vi "ArmMotorControl.vi"(2 "InputWhenFalse":dbl, 3 "EncoderDistance":dbl) -> ()   [LabVIEW 2018]
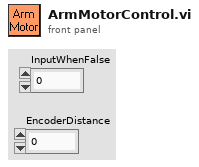
[diagram p1: front panel]
types:
  T1 = typedef "WPI_MotorControlDeviceRef.ctl" = cluster{"DeviceStatus":errorcluster, "Type":T2, "PWM":cluster{"PWM Channel":T3, "DeadBand":T4}, "CAN":cluster{"Device Number":u8, "SetOutput VI Ref":variant, "GetOutput VI Ref":variant, "Enable VI Ref":variant, "Disable VI Ref":variant, "Data":variant}, "Invert":bool, "DIO PWM":cluster{"PWM \"Enable\" Channel":T3, "DIOChannel":T5, "PWM Rate":dbl}}
  T2 = typedef "WPI_MotorControlType.ctl" = enum16{"PWM", "CAN", "DIO PWM"}
  T3 = typedef "FPGA_DIOPWMChannel.ctl" = enum8{"PWM 0", "PWM 1", "PWM 2", "PWM 3", "PWM 4", "PWM 5", "PWM 6", "PWM 7", "PWM 8", "PWM 9", "PWM MXP 0", "PWM MXP 1", "PWM MXP 2", "PWM MXP 3", "PWM MXP 4", "PWM MXP 5", "PWM MXP 6", "PWM MXP 7", "PWM MXP 8", "PWM MXP 9", "Invalid"}
  T4 = typedef "WPI_PWMDeadband.ctl" = cluster{"Name":string, "maxPositivePwm":i32, "minPositivePwm":i32, "centerPwm":i32, "maxNegativePwm":i32, "minNegativePwm":i32, "angularRange":u16}
  T5 = typedef "FPGA_DIOChannel.ctl" = enum8{"DIO 0", "DIO 1", "DIO 2", "DIO 3", "DIO 4", "DIO 5", "DIO 6", "DIO 7", "DIO 8", "DIO 9", "DIO MXP 0", "DIO MXP 1", "DIO MXP 2", "DIO MXP 3", "DIO MXP 4", "DIO MXP 5", "DIO MXP 6", "DIO MXP 7", "DIO MXP 8", "DIO MXP 9", "DIO MXP 10", "DIO MXP 11", "DIO MXP 12", "DIO MXP 13", "DIO MXP 14", "DIO MXP 15", "SPI Port CS1", "SPI Port CS2", "SPI Port CS3", "SPI Port MISO", "SPI Port MOSI", "Invalid"}
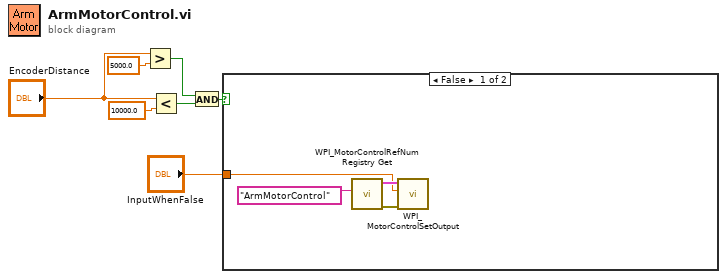
[diagram p0: block diagram]
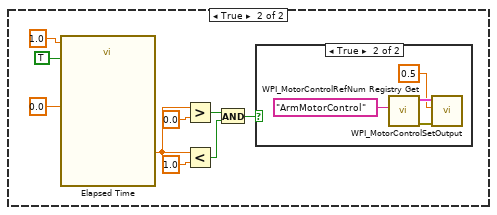
[diagram p2: hidden frame]
diagram:
  n1 = Greater?(x="EncoderDistance", y=5000.0) -> (0:w6:bool)
  n2 = Less?(x="EncoderDistance", y=10000.0) -> (x < y?=w5:bool)
  n3 = And(x=w6, y=w5) -> (x .and. y?=w7:bool)
  n4 = case shown="False" w7 {
    tunnel: "InputWhenFalse" -> [w8 _]
    frame False {
      n5 = call <vilib>:"WPI_MotorControlRefNum Registry Get.vi"("refnum name"="ArmMotorControl") -> ("error out"=w10:errorcluster, "MotorControlDevRef"=w9:T1)  [unwired: 9 in]
      n6 = call <vilib>:"WPI_MotorControlSetOutput.vi"("error in (no error)"=w10, "Output"=w8, "MotorControlDevRef"=w9) -> ()  [unwired: 6 in, 3 out]
    }
    frame True {
      n7 = call "Elapsed Time"("Time Target (s)"=1.0, "Reset"=TRUE ("Auto Reset"), "Set Start Time (s)"=0.0) -> ("Elapsed Time (s)"=w16:dbl)  [unwired: 9 in, 7 out]
      n8 = Greater?(x=w16, y=0.0) -> (0:w19:bool)
      n9 = Less?(x=w16, y=1.0) -> (x < y?=w20:bool)
      n10 = And(x=w19, y=w20) -> (x .and. y?=w18:bool)
      n11 = case shown="True" w18 {
        frame False {
        }
        frame True {
          n12 = call <vilib>:"WPI_MotorControlRefNum Registry Get.vi"("refnum name"="ArmMotorControl") -> ("error out"=w23:errorcluster, "MotorControlDevRef"=w24:T1)  [unwired: 9 in]
          n13 = call <vilib>:"WPI_MotorControlSetOutput.vi"("error in (no error)"=w23, "Output"=0.5, "MotorControlDevRef"=w24) -> ()  [unwired: 6 in, 3 out]
        }
      }
    }
  }
